vi "Initialise.vi"(2 "Que name":string, 5 "error in":errorcluster) -> (6 "error out":errorcluster)   [LabVIEW 2014, in "Que lib.lvlib"]
uses:
  Que lib.lvlib
  Controls/Queue cluster.ctl
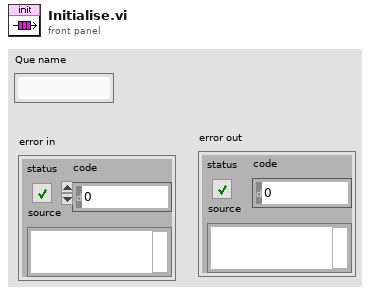
[diagram p1: front panel]
types:
  T1 = typedef "Que lib.lvlib/Queue cluster.ctl" = cluster{"Message":string, "Data":variant}
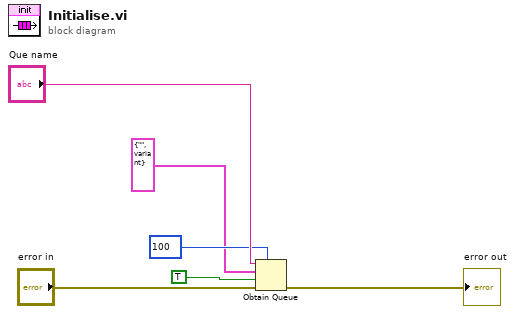
[diagram p0: block diagram]
diagram:
  n1 = Obtain Queue(max queue size (-1, unlimited)=100, name (unnamed)="Que name", element data type=T1 {"Message"="", "Data"=variant}, create if not found? (T)=TRUE, error in (no error)="error in") -> (error out=→"error out":errorcluster)  [unwired: 2 out]
